vi "AreaEnclosedDivided.vi"(10 "H":dbl[](array[numeric]), 11 "B":dbl[](array[numeric])) -> (0 "Done":bool, 3 "Area":dbl)   [LabVIEW 2019]
panel:
  out "error out":errorcluster
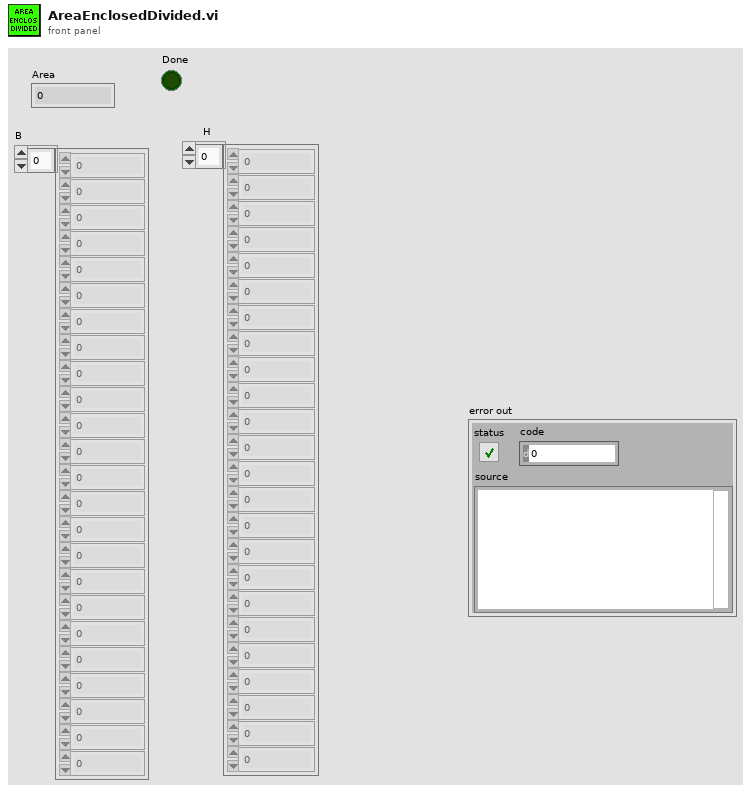
[diagram p1: front panel]
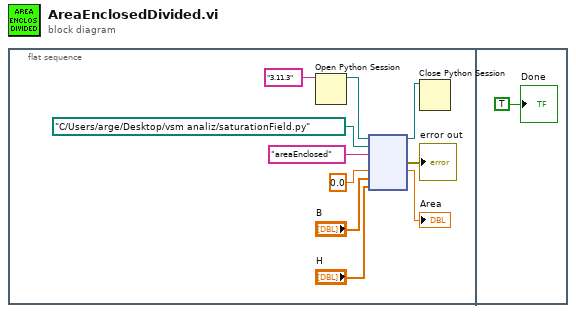
[diagram p0: block diagram]
diagram:
  n1 = flat-sequence {
    frame #0 {
      n2 = Open Python Session(python version="3.11.3" ("Python version")) -> (session out=w5:refnum<k35>)  [unwired: 2 in, 1 out]
      n3 = node(w5, path "C:/Users/arge/Desktop/vsm analiz/saturationField.py" ("module path"), "areaEnclosed" ("function name"), 0.0, "B", "H") -> (w7:refnum<k35>, →"error out":errorcluster, →"Area":dbl)  [unwired: 3 in, 2 out]
      n4 = Close Python Session(session in=w7) -> ()  [unwired: 1 in, 1 out]
    }
    frame #1 {
      "Done" <- TRUE ("Done")
    }
  }
